vi "Main.vi"() -> ()   [LabVIEW 2020]
doc: "Retrieves average CPU temp, if available. No warranty, use it at your own risk.\n\n© Aitor Solar, 2019.\nContact: aitor.solar@gmail.com"
uses:
  <vilib>/platform/TimedLoop/XDataNode/XDataNode.xnode
  <vilib>/Platform/TimedLoop/XDataNode/nitl_modes.ctl
  <vilib>/Platform/TimedLoop/XDataNode/XDNodeRunTimeDep.lvlib
  <vilib>/Platform/TimedLoop/XDataNode/wakeup.ctl
  <vilib>/Platform/TimedLoop/XDataNode/timing_clust.ctl
panel:
  in  "Read System Temps":bool
  out "Output Filename":path
  in  "Create New File":bool=TRUE
  in  "Accuracy Selector":enum16{"High Accuracy", "High Speed"}(ring)
  out "Waveform Chart":dynamicdata(graph)
  in  "stop":bool
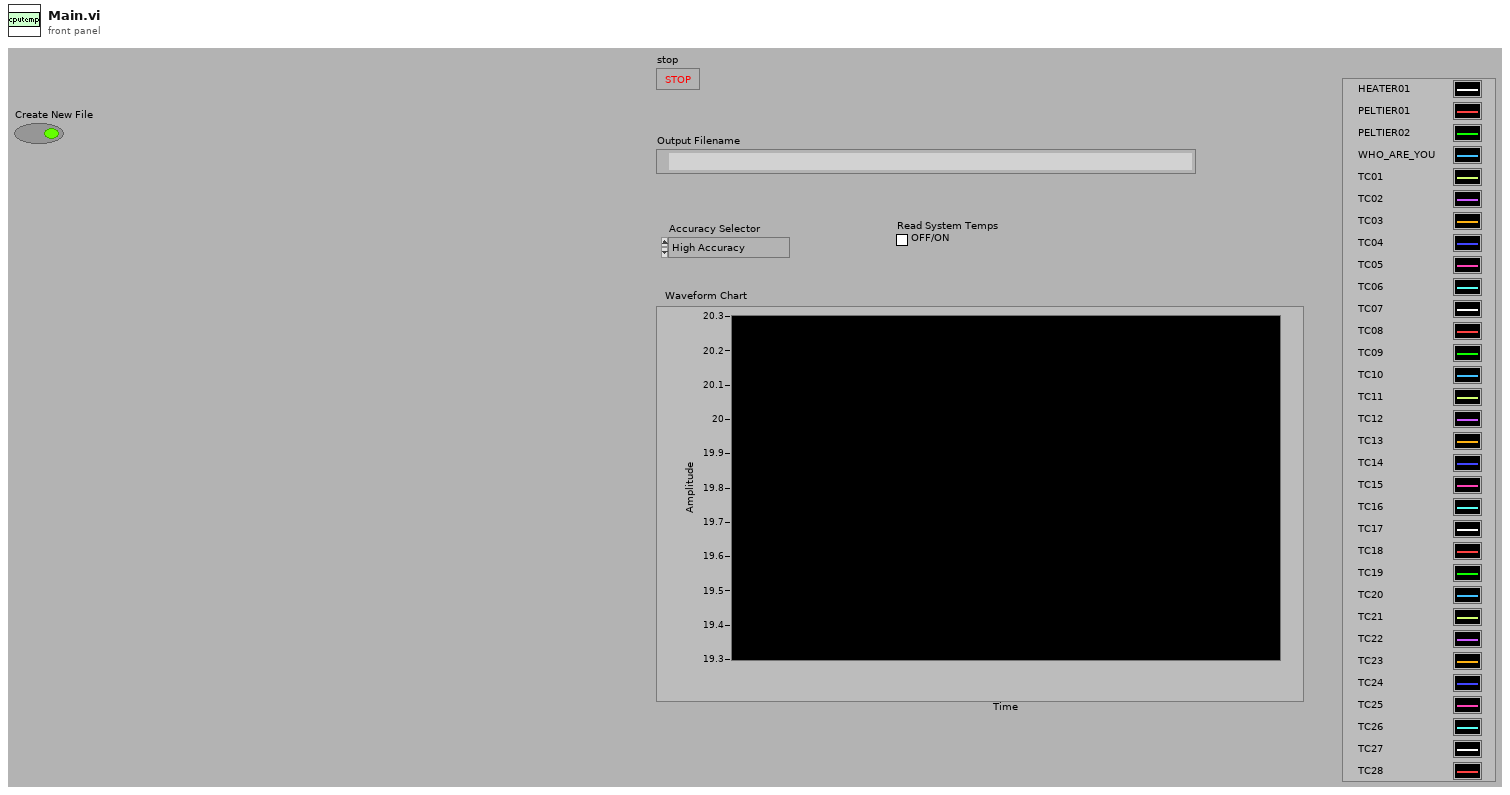
[diagram p1: front panel]
types:
  T1 = typedef "XDNodeRunTimeDep.lvlib/timing_clust.ctl" = cluster{"Expected End [f-1]":u64, "Actual End [f-1]":u64, "Finished Late? [f-1]":bool, "Expected End [i-1]":u64, "Actual End [i-1]":u64, "Finished Late? [i-1]":bool, "Expected Start [i]":u64, "Actual Start [i]":u64, "Expected Start [f]":u64, "Actual Start [f]":u64, "Source Name":string, "Structure Name":string, "Period":i64, "Deadline":i64, "Offset":i64, "Start":i64, "Priority":i32, "Timeout":i32, "Mode":T2, "Wakeup Reason":T3, "Error":errorcluster, "Source Type":string, "Secondary Source Type":string, "Global End Time":u64, "Global Start Time":u64, "Frame Duration":u64, "Iteration Duration":u64, "Assigned CPU":i32, "I/O Scan Engine Mode":u32}
  T2 = typedef "XDNodeRunTimeDep.lvlib/nitl_modes.ctl" = enum32{"No Change", "Process missed periods, maintain original phase", "Discard missed periods, maintain original phase", "Process missed periods, ignore original phase", "Discard missed periods, ignore original phase"}
  T3 = typedef "XDNodeRunTimeDep.lvlib/wakeup.ctl" = enum32{"Normal", "Aborted", "Asynchronous wakeup", "Timing source error", "Timed loop error", "Timeout"}
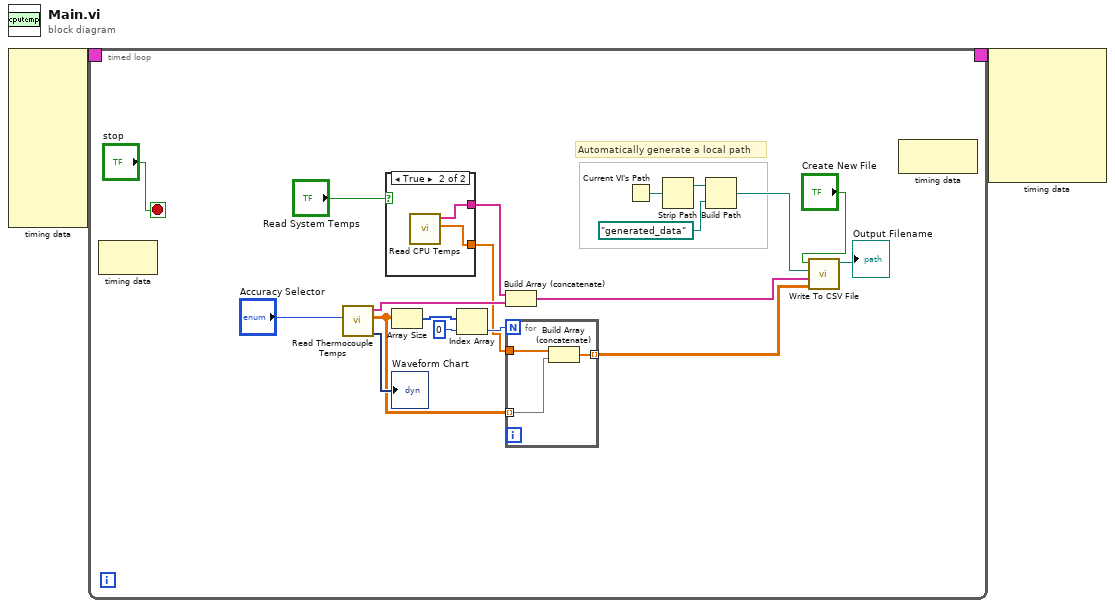
[diagram p0: block diagram]
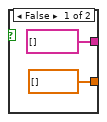
[diagram p2: hidden frame]
diagram:
  n1 = node-c288() -> (w2:T1)  [unwired: 10 in]
  n2 = timed-loop {
    timing: w2 -> [_]
    timing-out: [_] -> w1
    stop <- "stop" stop-if-true
    # "Automatically generate a local path"
    n3 = node-c288() -> ()  [unwired: 1 in, 1 out]
    n4 = call "Read Thermocouple Temps.vi"("Accuracy Selector"="Accuracy Selector") -> ("data"=→"Waveform Chart":dynamicdata, "Values"=w14:dbl[][], "Names"=w18:string[])  [unwired: 8 in]
    n5 = case shown="True" "Read System Temps" {
      tunnel: [string[] [] ("Names") w25] -> w9
      tunnel: [dbl[] [] ("Termperatures") w24] -> w8
      frame False {
      }
      frame True {
        n6 = call "Read CPU Temps.vi"() -> ("Termperatures"=w24:dbl[], "Names"=w25:string[])  [unwired: 9 in, 1 out]
      }
    }
    n7 = Array Size(array=w14) -> (size(s)=w17:i32[])
    n8 = Index Array(array=w17, index=0) -> (element=w15:i32)
    n9 = Build Array (concatenate)(w9, w18) -> (w12:string[])
    n10 = for {
      N: w15 -> [_]
      tunnel: w14 -> [w28] mode=indexing
      tunnel: w8 -> [w27]
      tunnel: [w26] -> w11 mode=indexing
      n11 = Build Array (concatenate)(w27, w28) -> (w26:dbl[])
    }
    n12 = Current VI's Path() -> (path=w6:path)
    n13 = Strip Path(path=w6) -> (stripped path=w5:path)  [unwired: 1 out]
    n14 = Build Path(base path=w5, name or relative path=path "generated_data") -> (appended path=w3:path)
    n15 = call "Write To CSV File.vi"("Values"=w11, "Names"=w12, "Output Directory"=w3, "Create New File"="Create New File") -> ("Output Filename"=→"Output Filename":path)  [unwired: 7 in]
    n16 = node-c288() -> ()  [unwired: 1 in, 1 out]
  }
  n17 = node-c288(w1) -> ()  [unwired: 7 out]
